vi "StartDrag.vi"(8 "error in (no error)":errorcluster, 10 "Coords":T1, 11 "OrderSelection in":refnum<class "OrderSelection.lvclass">) -> (0 "error out":errorcluster, 2 "InItem?":bool, 3 "OrderSelection out":refnum<class "OrderSelection.lvclass">)   [LabVIEW 2020, in "OrderSelection.lvclass"]
uses:
  OrderSelection.lvclass
  C:/Program Files/National Instruments/LabVIEW 2020/vi.lib/QSI/QControls/QControl Classes/GObject/GObject.lvclass
  C:/Program Files/National Instruments/LabVIEW 2020/vi.lib/QSI/QControls/QControl Classes/Picture/Picture.lvclass
  <vilib>/Utility/miscctls.llb/LVPoint32TypeDef.ctl
  Read ItemGraphic.vi
  Write SelectedItem.vi
panel:
  out "ItemBottom":i32
  out "ItemTop":i32
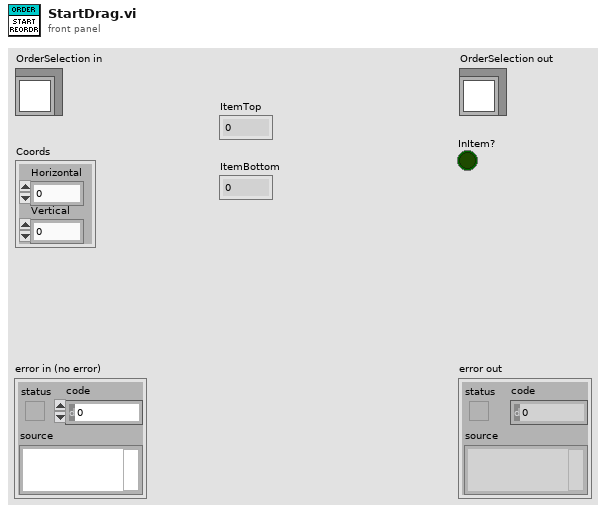
[diagram p1: front panel]
types:
  T1 = typedef "LVPoint32TypeDef.ctl" = cluster{"Horizontal":i32, "Vertical":i32}
  T2 = typedef "LVRectTypeDef.ctl" = cluster{"Left":i16, "Top":i16, "Right":i16, "Bottom":i16}
  T3 = typedef "imagedata.ctl" = cluster{"image type":i32, "image depth":i32, "image":u8[], "mask":u8[], "colors":u32[], "Rectangle":cluster{"left":i16, "top":i16, "right":i16, "bottom":i16}}
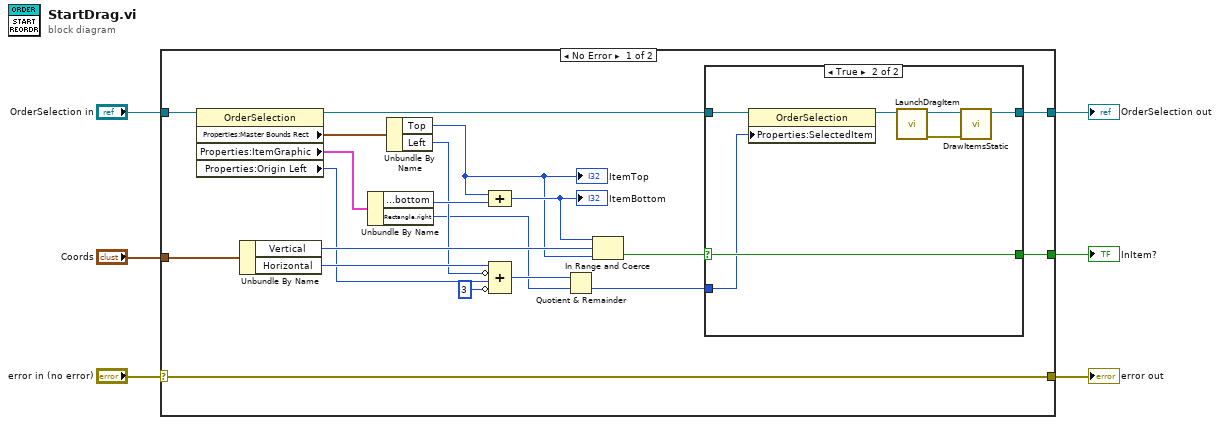
[diagram p0: block diagram]
diagram:
  n1 = case shown="No Error" "error in (no error)" {
    selector: "error in (no error)" -> [w25 w37]
    tunnel: [w25 w37] -> w5
    tunnel: [w10 w36] -> w3
    tunnel: "OrderSelection in" -> [w26 w36]
    tunnel: "Coords" -> [w21 _]
    tunnel: [w8 _] -> w1
    frame No Error {
      n2 = property class="OrderSelection"(reference=w26) -> (reference out=w11:refnum<class "OrderSelection.lvclass">, "Properties:Master Bounds Rect"=w23:T2, "Properties:ItemGraphic"=w24:T3, "Properties:Origin Left"=w13:i16)  [unwired: 1 in, 1 out]
      n3 = Unbundle By Name(w21) -> ("Vertical"=w19:i32, "Horizontal"=w18:i32)
      n4 = Unbundle By Name(w24) -> ("Rectangle.bottom"=w22:i16, "Rectangle.right"=w15:i16)
      n5 = Unbundle By Name(w23) -> ("Top"=w14:i16, "Left"=w17:i16)
      "ItemTop" <- w14
      n6 = Compound Arithmetic op=ADD(w14, w22) -> (w20:i16)
      "ItemBottom" <- w20
      n7 = Compound Arithmetic op=ADD(w18, invert w17, w13, invert i16 3 ("value")) -> (w16:i32)
      n8 = Quotient & Remainder(x=w16, y=w15) -> (floor(x/y)=w7:i32)  [unwired: 1 out]
      n9 = In Range and Coerce(upper limit=w20, x=w19, lower limit=w14) -> (In Range?=w9:bool)  [unwired: 1 out]
      n10 = case shown="True" w9 {
        selector: w9 -> [w27 w35]
        tunnel: w11 -> [w28 w34]
        tunnel: [w28 w30] -> w10
        tunnel: [w27 w35] -> w8
        tunnel: w7 -> [_ w32]
        frame False {
        }
        frame True {
          n11 = property class="OrderSelection"(reference=w34, "Properties:SelectedItem"=w32) -> (reference out=w33:refnum<class "OrderSelection.lvclass">)  [unwired: 1 in, 1 out]
          n12 = call "LaunchDragItem.vi"("OrderSelection in"=w33) -> ("error out"=w29:errorcluster, "OrderSelection out"=w31:refnum<class "OrderSelection.lvclass">)  [unwired: 9 in]
          n13 = call "DrawItemsStatic.vi"("error in (no error)"=w29, "OrderSelection in"=w31) -> ("OrderSelection out"=w30:refnum<class "OrderSelection.lvclass">)  [unwired: 8 in, 1 out]
        }
      }
    }
    frame Error {
    }
  }
  "error out" <- w5
  "OrderSelection out" <- w3
  "InItem?" <- w1
